vi "Create Build Trigger Cron String.vi"(11 "Cron":T1={"Day of Week"=enum."Sunday", "Hour"=1, "Enable?"=FALSE} {"Hour" min=0 max=23}) -> (3 "String":string)   [LabVIEW 2014]
uses:
  Controls/Cron String - STYP.ctl
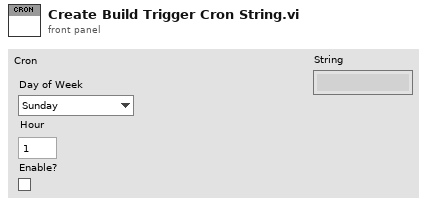
[diagram p1: front panel]
types:
  T1 = typedef "Cron String - STYP.ctl" = cluster{"Day of Week":enum16{"Everyday", "Sunday", "Monday", "Tuesday", "Wednesday", "Thursday", "Friday", "Saturday"}, "Hour":i32, "Enable?":bool}
  T2 = enum16{"Everyday", "Sunday", "Monday", "Tuesday", "Wednesday", "Thursday", "Friday", "Saturday"}
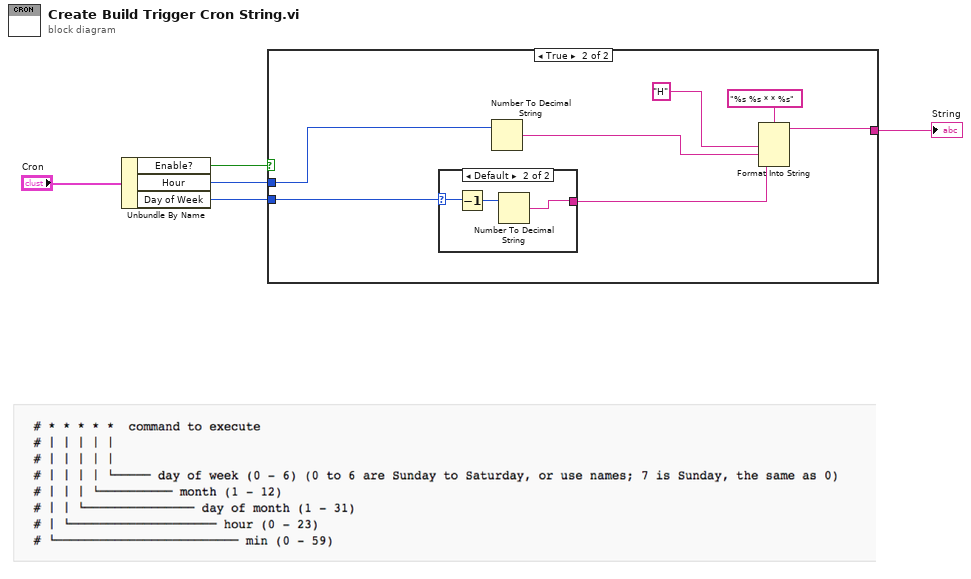
[diagram p0: block diagram]
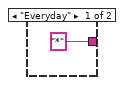
[diagram p3: hidden frame]
diagram:
  n1 = Unbundle By Name("Cron") -> ("Enable?"=w1:bool, "Hour"=w3:i32, "Day of Week"=w4:T2)
  n2 = case shown="True" w1 {
    tunnel: w4 -> [_ w12]
    tunnel: w3 -> [_ w9]
    tunnel: [_ w7] -> w2
    frame False {
    }
    frame True {
      n3 = case shown="Default" w12 {
        selector: w12 -> [_ w16]
        tunnel: ["*" w14] -> w10
        frame "Everyday" {
        }
        frame Default {
          n4 = Decrement(x=w16) -> (x-1=w15:T2)
          n5 = Number To Decimal String(number=w15) -> (decimal integer string=w14:string)  [unwired: 1 in]
        }
      }
      n6 = Number To Decimal String(number=w9) -> (decimal integer string=w8:string)  [unwired: 1 in]
      n7 = Format Into String(format string="%s %s * * %s", "H" ("input 1"), w8, w10) -> (resulting string=w7:string)  [unwired: 2 in, 1 out]
    }
  }
  "String" <- w2
